vi "LED_ctrl_subVI.vi"(2 "stop":bool, 3 "error in (no error)":errorcluster, 4 "Numeric in":dbl) -> (0 "HOT\nSurface":bool, 1 "error out":errorcluster)   [LabVIEW 2021]
uses:
  <vilib>/myRIO/Instrument Drivers/Onboard IO/PWM/typedefs/PWM Reference.ctl
  <vilib>/myRIO/Common/Instrument Driver Framework/Utilities/typedefs/myRIO Generic Hardware Reference.ctl
  <vilib>/myRIO/Common/Instrument Driver Framework/Utilities/typedefs/Hardware Version Enum.ctl
  <vilib>/myRIO/Common/Instrument Driver Framework/Utilities/typedefs/myRIO v1.0 Reference.ctl
  <vilib>/myRIO/Common/Instrument Driver Framework/Utilities/typedefs/Generic FPGA Reference.ctl
  <vilib>/myRIO/Common/Instrument Driver Framework/myRIO v1.0/PWM/typedefs/PWM Channels Enum.ctl
  <vilib>/myRIO/Instrument Drivers/Onboard IO/PWM/typedefs/PWM Configuration.ctl
  <vilib>/userDefined/High Color/nirio_resource_hc.ctl
  <vilib>/myRIO/Common/Instrument Driver Framework/Utilities/vis/Is FPGA Ref Available.vi
  <vilib>/myRIO/Common/Instrument Driver Framework/myRIO v1.0/PWM/vis/myRIO v1.1 Open PWM.vi
  <vilib>/myRIO/Instrument Drivers/Onboard IO/PWM/vis/Set Duty Cycle and Frequency.vi
  <vilib>/myRIO/Common/Instrument Driver Framework/Utilities/vis/Validate Channels.vi
  <vilib>/myRIO/Common/Instrument Driver Framework/myRIO v1.0/PWM/vis/myRIO v1.0 Reserve PWM.vi
  <vilib>/myRIO/Common/Instrument Driver Framework/myRIO v1.0/PWM/vis/myRIO v1.0 Build MUX Configuration PWM.vi
  <vilib>/myRIO/Common/Instrument Driver Framework/myRIO v1.0/Resource Manager/vis/myRIO v1.0 Reserve Channel List.vi
  <vilib>/myRIO/Common/Instrument Driver Framework/myRIO v1.0/Resource Manager/vis/myRIO v1.0 Create Configuration List.vi
  <vilib>/myRIO/Common/Instrument Driver Framework/myRIO v1.0/Resource Manager/vis/myRIO v1.0 Reserve Channel.vi
  <vilib>/myRIO/Common/Instrument Driver Framework/myRIO v1.0/Resource Manager/vis/myRIO v1.0 Unreserve Channel.vi
  <vilib>/myRIO/Common/Instrument Driver Framework/myRIO v1.0/Resource Manager/vis/myRIO v1.0 Build Mutex Name.vi
  <vilib>/Utility/VariantDataType/GetNumericInfo.vi
  <vilib>/Utility/error.llb/Error Cluster From Error Code.vi
  <vilib>/myRIO/Common/Instrument Driver Framework/myRIO v1.0/myRIO v1.1 Open.vi
  <vilib>/myRIO/Common/Instrument Driver Framework/Utilities/vis/IO Manager.vi
  <vilib>/myRIO/Common/Instrument Driver Framework/Utilities/vis/Configuration Manager.vi
  <vilib>/myRIO/Common/Instrument Driver Framework/myRIO v1.0/Resource Manager/vis/myRIO v1.0 Configure IO.vi
  <vilib>/myRIO/Common/Instrument Driver Framework/myRIO v1.0/myRIO v1.0 Close.vi
  <vilib>/myRIO/Common/Instrument Driver Framework/myRIO v1.0/PWM/vis/myRIO v1.0 Write PWM.vi
  <vilib>/myRIO/Express VI/Onboard IO/PWM/PWM Express VI.xnode
  <vilib>/myRIO/Instrument Drivers/Onboard IO/PWM/vis/myRIO PWM Open.xnode
  <vilib>/myRIO/Instrument Drivers/Onboard IO/PWM/PWM.lvlib
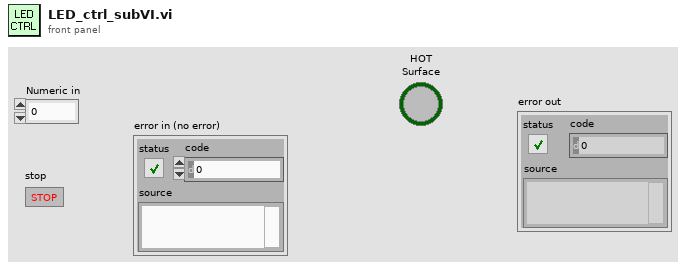
[diagram p1: front panel]
types:
  T1 = typedef "PWM.lvlib/PWM Reference.ctl" = cluster{"myRIO Reference":T2, "PWM Channels Enum":T6, "PWM Configuration":T7}
  T2 = typedef "myRIO Generic Hardware Reference.ctl" = cluster{"myRIO Model":T3, "myRIO Hardware Reference":T4}
  T3 = typedef "Hardware Version Enum.ctl" = enum16{"Unknown", "myRIO-1900", "myRIO-1950", "roboRIO", "NI ELVIS RIO CM", "ELVIS III"}
  T4 = typedef "myRIO v1.0 Reference.ctl" = cluster{"Generic FPGA Reference":T5, "Allow multiple opens":bool}
  T5 = typedef "Generic FPGA Reference.ctl" = refnum<k20>
  T6 = typedef "PWM Channels Enum.ctl" = enum16{"Not Connected", "C/PWM0", "C/PWM1", "A/PWM0", "A/PWM1", "A/PWM2", "A/PWM3", "A/PWM4", "A/PWM5", "A/PWM6", "A/PWM7", "A/PWM8", "A/PWM9", "A/PWM10", "A/PWM11", "A/PWM12", "A/PWM13", "A/PWM14", "A/PWM15", "A/PWM16", "A/PWM17", "A/PWM18", "A/PWM19", "B/PWM0", "B/PWM1", "B/PWM2", "B/PWM3", "B/PWM4", "B/PWM5", "B/PWM6", "B/PWM7", "B/PWM8", "B/PWM9", "B/PWM10", "B/PWM11", "B/PWM12", "B/PWM13", "B/PWM14", "B/PWM15", "B/PWM16", "B/PWM17", "B/PWM18", "B/PWM19", "PWM/PWM0", "PWM/PWM1", "PWM/PWM2", "PWM/PWM3", "PWM/PWM4", "PWM/PWM5", "PWM/PWM6", "PWM/PWM7", "PWM/PWM8", "PWM/PWM9"}
  T7 = typedef "PWM.lvlib/PWM Configuration.ctl" = cluster{"Frequency":dbl, "Duty Cycle":dbl}
  T8 = typedef "nirio_resource_hc.ctl" = tag
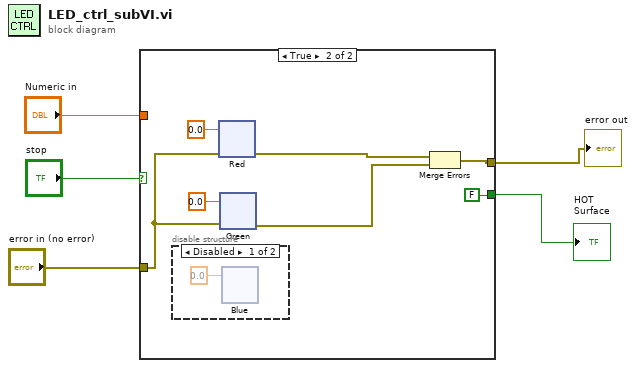
[diagram p0: block diagram]
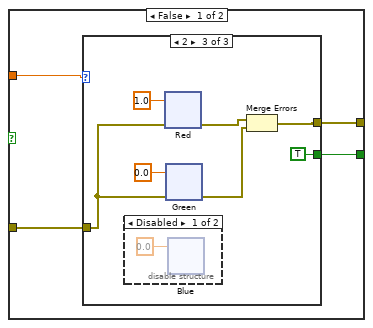
[diagram p2: hidden frame]
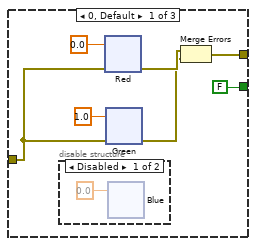
[diagram p3: hidden frame]
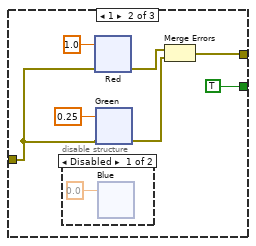
[diagram p5: hidden frame]
diagram:
  n1 = case shown="True" "stop" {
    tunnel: "Numeric in" -> [w9 _]
    tunnel: [w8 FALSE] -> w3
    tunnel: "error in (no error)" -> [w7 w352]
    tunnel: [w6 w349] -> w1
    frame False {
      n2 = case shown="2" w9 {
        tunnel: [FALSE TRUE ("HOT\nSurface") TRUE] -> w8
        tunnel: w7 -> [w13 w126 w239]
        tunnel: [w10 w123 w236] -> w6
        frame 0, Default {
          n3 = disable-structure shown="Disabled" {
            frame Disabled {
              n4 = xnode "Blue"("Duty Cycle"=0.0) -> ()  [unwired: 1 in, 1 out]
            }
            frame Enabled {
            }
          }
          n5 = xnode "Red"("error in (no error)"=w13, "Duty Cycle"=0.0) -> ("error out"=w12:errorcluster)
          n6 = xnode "Green"("error in (no error)"=w13, "Duty Cycle"=1.0) -> ("error out"=w11:errorcluster)
          n7 = Merge Errors(w12, w11) -> (w10:errorcluster)
        }
        frame 1 {
          n8 = disable-structure shown="Disabled" {
            frame Disabled {
              n9 = xnode "Blue"("Duty Cycle"=0.0) -> ()  [unwired: 1 in, 1 out]
            }
            frame Enabled {
            }
          }
          n10 = xnode "Red"("error in (no error)"=w126, "Duty Cycle"=1.0) -> ("error out"=w124:errorcluster)
          n11 = xnode "Green"("error in (no error)"=w126, "Duty Cycle"=0.25) -> ("error out"=w125:errorcluster)
          n12 = Merge Errors(w124, w125) -> (w123:errorcluster)
        }
        frame 2 {
          n13 = disable-structure shown="Disabled" {
            frame Disabled {
              n14 = xnode "Blue"("Duty Cycle"=0.0) -> ()  [unwired: 1 in, 1 out]
            }
            frame Enabled {
            }
          }
          n15 = xnode "Red"("error in (no error)"=w239, "Duty Cycle"=1.0) -> ("error out"=w238:errorcluster)
          n16 = xnode "Green"("error in (no error)"=w239, "Duty Cycle"=0.0) -> ("error out"=w237:errorcluster)
          n17 = Merge Errors(w238, w237) -> (w236:errorcluster)
        }
      }
    }
    frame True {
      n18 = disable-structure shown="Disabled" {
        frame Disabled {
          n19 = xnode "Blue"("Duty Cycle"=0.0) -> ()  [unwired: 1 in, 1 out]
        }
        frame Enabled {
        }
      }
      n20 = xnode "Red"("error in (no error)"=w352, "Duty Cycle"=0.0) -> ("error out"=w350:errorcluster)
      n21 = xnode "Green"("error in (no error)"=w352, "Duty Cycle"=0.0) -> ("error out"=w351:errorcluster)
      n22 = Merge Errors(w350, w351) -> (w349:errorcluster)
    }
  }
  "HOT\nSurface" <- w3
  "error out" <- w1
